vi "Autonomous Independent.vi"   [LabVIEW 2020]
doc: "This VI is called when autonomous begins, and will automatically be terminated when autonomous ends. You can carry out timed or sensor driven robot movement independently without needing to return to the caller."
uses:
  <vilib>/Rock Robotics/WPI/ThirdParty/Phoenix-LabVIEW/Motor Controller/Controls/CTRE_Phoenix_MotorControl_ControlMode.ctl
  <vilib>/Rock Robotics/WPI/Solenoid/WPI_SolenoidValue.ctl
  <vilib>/Rock Robotics/Network Tables/NT Read String.vi
  <vilib>/Rock Robotics/WPI/Utilities/WPI_GetSetVariantRefNum.vi
  <vilib>/Rock Robotics/WPI/RobotDrive/WPI_RobotDriveArcadeDrive_Standard(NoSaturation).vi
  <vilib>/Rock Robotics/WPI/Solenoid/WPI_SolenoidSetEnum.vi
  <vilib>/Rock Robotics/Network Tables/NT Read Number.vi
panel:
  # "Be sure to right-click and choose Data Operations>>Make Current Value default if you want to save the array values with the VI"
types:
  T1 = typedef "WPI_RobotDriveDevRef.ctl" = cluster{"DevStatus":errorcluster, "Motors[]":T2[], "Square Inputs":bool, "Max Output":dbl}
  T2 = typedef "WPI_MotorControlDeviceRef.ctl" = cluster{"DeviceStatus":errorcluster, "Type":T3, "PWM":cluster{"PWM Channel":T4, "DeadBand":T5}, "CAN":cluster{"Device Number":u8, "SetOutput VI Ref":variant, "GetOutput VI Ref":variant, "Enable VI Ref":variant, "Disable VI Ref":variant, "Data":variant}, "Invert":bool, "DIO PWM":cluster{"PWM \"Enable\" Channel":T4, "DIOChannel":T6, "PWM Rate":dbl}}
  T3 = typedef "WPI_MotorControlType.ctl" = enum16{"PWM", "CAN", "DIO PWM"}
  T4 = typedef "FPGA_DIOPWMChannel.ctl" = enum8{"PWM 0", "PWM 1", "PWM 2", "PWM 3", "PWM 4", "PWM 5", "PWM 6", "PWM 7", "PWM 8", "PWM 9", "PWM MXP 0", "PWM MXP 1", "PWM MXP 2", "PWM MXP 3", "PWM MXP 4", "PWM MXP 5", "PWM MXP 6", "PWM MXP 7", "PWM MXP 8", "PWM MXP 9", "Invalid"}
  T5 = typedef "WPI_PWMDeadband.ctl" = cluster{"Name":string, "maxPositivePwm":i32, "minPositivePwm":i32, "centerPwm":i32, "maxNegativePwm":i32, "minNegativePwm":i32, "angularRange":u16}
  T6 = typedef "FPGA_DIOChannel.ctl" = enum8{"DIO 0", "DIO 1", "DIO 2", "DIO 3", "DIO 4", "DIO 5", "DIO 6", "DIO 7", "DIO 8", "DIO 9", "DIO MXP 0", "DIO MXP 1", "DIO MXP 2", "DIO MXP 3", "DIO MXP 4", "DIO MXP 5", "DIO MXP 6", "DIO MXP 7", "DIO MXP 8", "DIO MXP 9", "DIO MXP 10", "DIO MXP 11", "DIO MXP 12", "DIO MXP 13", "DIO MXP 14", "DIO MXP 15", "SPI Port CS1", "SPI Port CS2", "SPI Port CS3", "SPI Port MISO", "SPI Port MOSI", "Invalid"}
  T7 = typedef "WPI_SolenoidDevRef.ctl" = cluster{"DevStatus":errorcluster, "Pneumatics Control Module":u8, "Forward Solenoid Channel":T8, "Reverse Solenoid Channel":T8}
  T8 = typedef "WPI_SolenoidChannel.ctl" = enum8{"Solenoid 0", "Solenoid 1", "Solenoid 2", "Solenoid 3", "Solenoid 4", "Solenoid 5", "Solenoid 6", "Solenoid 7", "Solenoid 8", "Solenoid 9", "Solenoid 10", "Solenoid 11", "Solenoid 12", "Solenoid 13", "Solenoid 14", "Solenoid 15", "Invalid"}
  T9 = typedef "WPI_SolenoidValue.ctl" = enum16{"Off", "On", "Forward", "Reverse"}
  T10 = typedef "CTRE_Phoenix_MotorControl_ControlMode.ctl" = u16
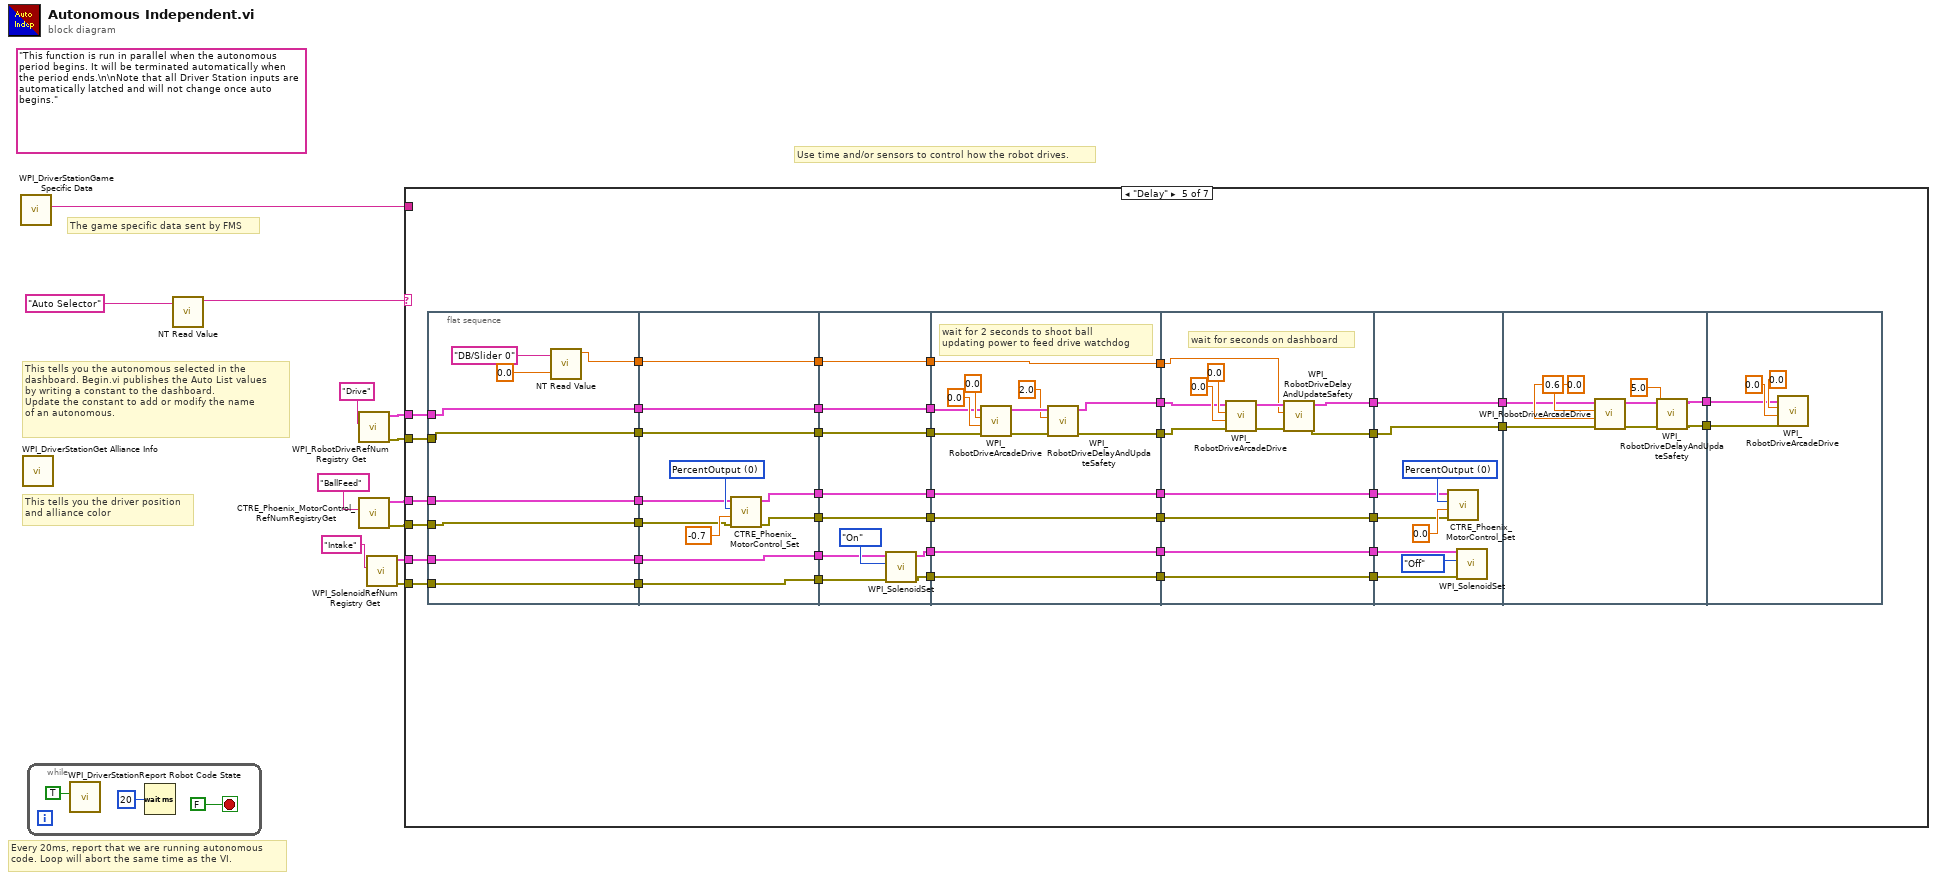
[diagram p0: block diagram]
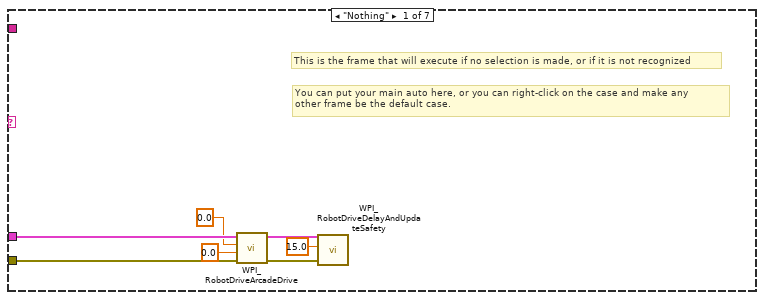
[diagram p2: hidden frame]
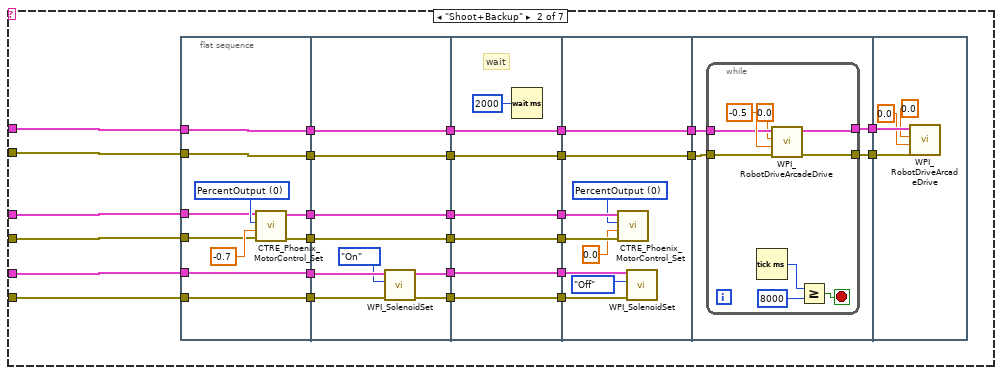
[diagram p3: hidden frame]
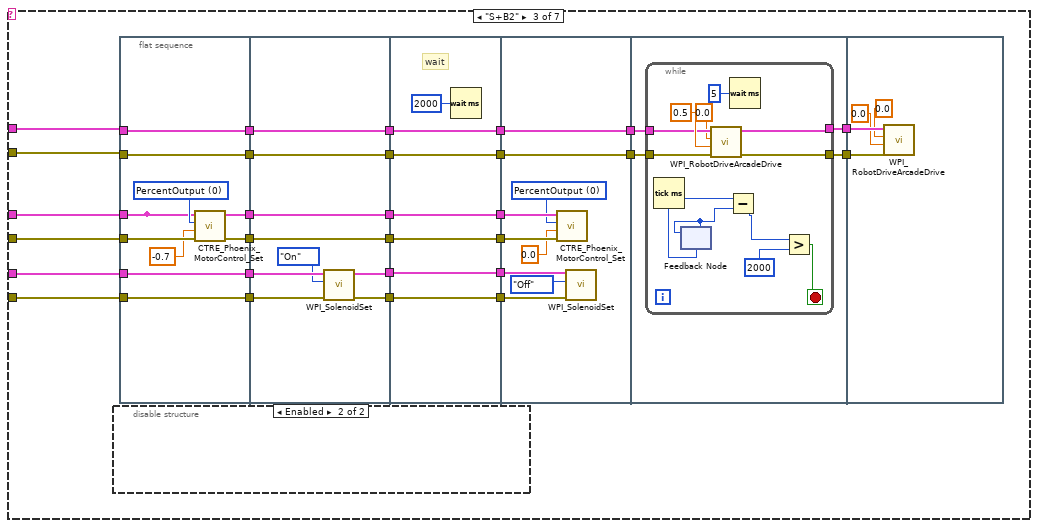
[diagram p4: hidden frame]
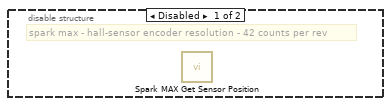
[diagram p5: hidden frame]
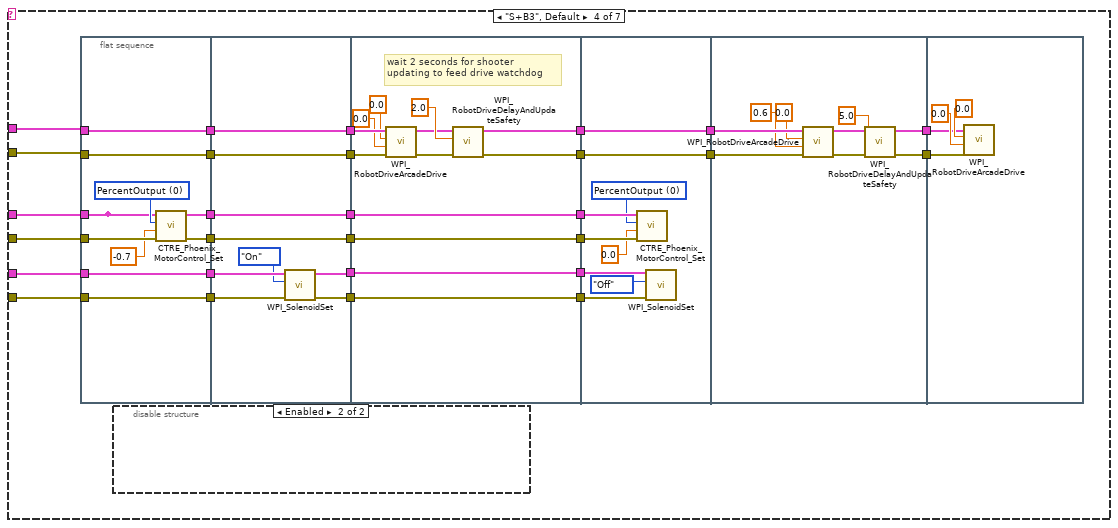
[diagram p6: hidden frame]
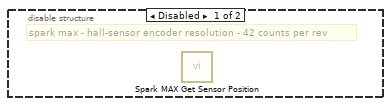
[diagram p7: hidden frame]
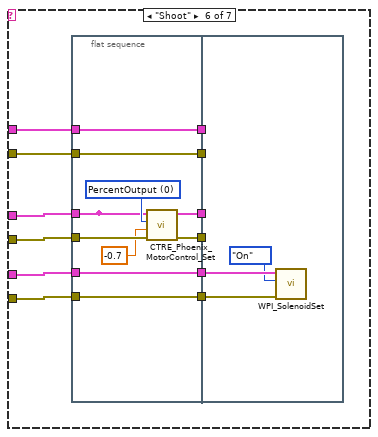
[diagram p8: hidden frame]
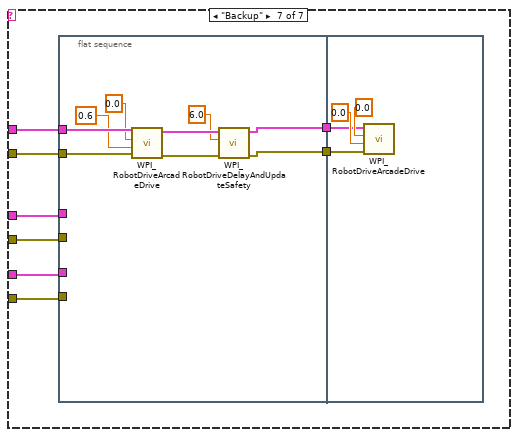
[diagram p9: hidden frame]
diagram:
  (unwired) "This function is run in parallel when the autonomous period begins. It will be terminated automatically when the period ends.\n\nNote that all Driver Station inputs are automatically latched and will not change once auto begins."
  # "The game specific data sent by FMS"
  # "This tells you the autonomous selected in the \ndashboard. Begin.vi publishes the Auto List values\nby writing a constant to the dashboard.\nUpdate the constant to add or modify the name\nof an autonomous."
  # "Every 20ms, report that we are running autonomous\ncode. Loop will abort the same time as the VI."
  # "Use time and/or sensors to control how the robot drives."
  # "This tells you the driver position\nand alliance color"
  n1 = call <vilib>:"WPI_DriverStationGame Specific Data.vi"() -> ("Game Specific Data"=w10:string)  [unwired: 11 in]
  n2 = call <vilib>:"WPI_DriverStationGet Alliance Info.vi"() -> ()  [unwired: 12 out]
  n3 = while {
    stop <- FALSE stop-if-true
    n4 = call <vilib>:"WPI_DriverStationReport Robot Code State.vi"("Autonomous"=TRUE) -> ()  [unwired: 10 in, 1 out]
    n5 = Wait (ms)(milliseconds to wait=u32 20) -> ()  [unwired: 1 out]
  }
  n6 = call-poly <vilib>:"NT Read Value.vi"("Name"="Auto Selector") -> ("String"=w11:string)  [unwired: 9 in, 1 out]
  n7 = call <vilib>:"WPI_RobotDriveRefNum Registry Get.vi"("refnum name"="Drive") -> ("error out"=w8:errorcluster, "RobotDriveDevRef"=w7:T1)  [unwired: 9 in]
  n8 = call <vilib>:"CTRE_Phoenix_MotorControl_RefNumRegistryGet.vi"("refnum name"="BallFeed") -> ("error out"=w2:errorcluster, "PhoenixMotorControlDevRef"=w1:T2)  [unwired: 9 in]
  n9 = call <vilib>:"WPI_SolenoidRefNum Registry Get.vi"("refnum name"="Intake") -> ("error out"=w4:errorcluster, "SolenoidDevRef"=w3:T7)  [unwired: 9 in]
  n10 = case shown="\"Delay\"" w11 {
    tunnel: w10 -> [_ _ _ _ _ _ _]
    tunnel: w8 -> [w21 w36 w107 w192 w294 w395 w422]
    tunnel: w7 -> [w22 w31 w108 w193 w301 w396 w423]
    tunnel: w4 -> [_ w26 w103 w188 w303 w391 w418]
    tunnel: w3 -> [_ w25 w104 w189 w306 w392 w419]
    tunnel: w2 -> [_ w24 w105 w190 w309 w393 w420]
    tunnel: w1 -> [_ w23 w106 w191 w310 w394 w421]
    frame "Nothing" {
      # "You can put your main auto here, or you can right-click on the case and make any\nother frame be the default case."
      # "This is the frame that will execute if no selection is made, or if it is not recognized"
      n11 = call-poly <vilib>:"WPI_RobotDriveArcadeDrive.vi"("error in (no error)"=w21, "Y axis value"=0.0, "X axis value"=0.0, "RobotDriveDevRef"=w22) -> ("error out"=w19:errorcluster, "RobotDriveDevRef"=w20:T1)  [unwired: 5 in, 1 out]
      n12 = call <vilib>:"WPI_RobotDriveDelayAndUpdateSafety.vi"("error in (no error)"=w19, "Delay (s)"=15.0, "RobotDriveDevRef"=w20) -> ()  [unwired: 7 in, 2 out]
    }
    frame "Shoot+Backup" {
      n13 = flat-sequence {
        tunnel: [w53] -> w50
        tunnel: [w54] -> w49
        tunnel: [w58] -> w46
        tunnel: [w57] -> w39
        tunnel: w36 -> [w56]
        tunnel: [w56] -> w35
        tunnel: w31 -> [w55]
        tunnel: [w55] -> w30
        tunnel: w26 -> [w54]
        tunnel: w25 -> [w53]
        tunnel: w24 -> [w52]
        tunnel: w23 -> [w51]
        tunnel: w50 -> [w69]
        tunnel: w49 -> [w68]
        tunnel: [w66] -> w47
        tunnel: w46 -> [w66]
        tunnel: [w65] -> w44
        tunnel: [w64] -> w42
        tunnel: [w63] -> w40
        tunnel: w39 -> [w63]
        tunnel: w35 -> [w62]
        tunnel: [w62] -> w34
        tunnel: w30 -> [w61]
        tunnel: [w61] -> w27
        tunnel: [w75] -> w48
        tunnel: w47 -> [w75]
        tunnel: [w74] -> w45
        tunnel: w44 -> [w74]
        tunnel: [w73] -> w43
        tunnel: w42 -> [w73]
        tunnel: [w72] -> w41
        tunnel: w40 -> [w72]
        tunnel: w34 -> [w71]
        tunnel: [w71] -> w32
        tunnel: [w70] -> w28
        tunnel: w27 -> [w70]
        tunnel: w48 -> [w85]
        tunnel: w45 -> [w83]
        tunnel: w43 -> [w84]
        tunnel: w41 -> [w82]
        tunnel: [w78] -> w33
        tunnel: w32 -> [w78]
        tunnel: [w77] -> w29
        tunnel: w28 -> [w77]
        tunnel: [w89] -> w38
        tunnel: [w88] -> w37
        tunnel: w33 -> [w87]
        tunnel: w29 -> [w86]
        tunnel: w38 -> [w102]
        tunnel: w37 -> [w101]
        frame #0 {
          w60 = T10 0 items=["PercentOutput"=0, "Position"=1, "Velocity"=2, "Current"=3, "Follower"=5, "MotionProfile"=6, "MotionMagic"=7, "MotionProfileArc"=10, "Disabled"=15] ("Control Mode")
          n14 = call <vilib>:"CTRE_Phoenix_MotorControl_Set.vi"("error in (no error)"=w52, "Output"=-0.7, "Control Mode"=w60, "PhoenixMotorControlDevRef"=w51) -> ("error out"=w57:errorcluster, "PhoenixMotorControlDevRef"=w58:T2)  [unwired: 6 in]
        }
        frame #1 {
          n15 = call-poly <vilib>:"WPI_SolenoidSet.vi"("error in (no error)"=w68, "Value"=WPI_SolenoidValue."On", "SolenoidDevRef"=w69) -> ("error out"=w64:errorcluster, "SolenoidDevRef"=w65:T7)  [unwired: 7 in]
        }
        frame #2 {
          # "wait"
          n16 = Wait (ms)(milliseconds to wait=u32 2000) -> ()  [unwired: 1 out]
        }
        frame #3 {
          w81 = T10 0 items=["PercentOutput"=0, "Position"=1, "Velocity"=2, "Current"=3, "Follower"=5, "MotionProfile"=6, "MotionMagic"=7, "MotionProfileArc"=10, "Disabled"=15] ("Control Mode")
          n17 = call <vilib>:"CTRE_Phoenix_MotorControl_Set.vi"("error in (no error)"=w82, "Output"=0.0, "Control Mode"=w81, "PhoenixMotorControlDevRef"=w85) -> ()  [unwired: 6 in, 2 out]
          n18 = call-poly <vilib>:"WPI_SolenoidSet.vi"("error in (no error)"=w84, "Value"=WPI_SolenoidValue."Off", "SolenoidDevRef"=w83) -> ()  [unwired: 7 in, 2 out]
        }
        frame #4 {
          n19 = while {
            tunnel: w86 -> [w94]
            tunnel: w87 -> [w93]
            tunnel: [w91] -> w89
            tunnel: [w90] -> w88
            stop <- w98 stop-if-true
            n20 = Tick Count (ms)() -> (millisecond timer value=w97:u32)
            n21 = call-poly <vilib>:"WPI_RobotDriveArcadeDrive.vi"("error in (no error)"=w93, "Y axis value"=-0.5, "X axis value"=0.0, "RobotDriveDevRef"=w94) -> ("error out"=w90:errorcluster, "RobotDriveDevRef"=w91:T1)  [unwired: 5 in, 1 out]
            n22 = Greater Or Equal?(x=w97, y=u32 8000) -> (x >= y?=w98:bool)
          }
        }
        frame #5 {
          n23 = call-poly <vilib>:"WPI_RobotDriveArcadeDrive.vi"("error in (no error)"=w101, "Y axis value"=0.0, "X axis value"=0.0, "RobotDriveDevRef"=w102) -> ()  [unwired: 5 in, 3 out]
        }
      }
    }
    frame "S+B2" {
      n24 = disable-structure shown="Enabled" {
        frame Disabled {
          # "spark max - hall-sensor encoder resolution - 42 counts per rev"
          n25 = call <vilib>:"Spark MAX Get Sensor Position.vi"() -> ()  [unwired: 8 in, 4 out]
        }
        frame Enabled {
        }
      }
      n26 = flat-sequence {
        tunnel: [w131] -> _
        tunnel: w105 -> [w140]
        tunnel: [w137] -> w130
        tunnel: w104 -> [w137]
        tunnel: [w136] -> w129
        tunnel: w103 -> [w136]
        tunnel: [w135] -> w128
        tunnel: [w134] -> w127
        tunnel: [w133] -> w126
        tunnel: w108 -> [w133]
        tunnel: [w132] -> w125
        tunnel: w107 -> [w132]
        tunnel: w106 -> [w131]
        tunnel: w130 -> [w149]
        tunnel: w129 -> [w148]
        tunnel: [w146] -> w124
        tunnel: w128 -> [w146]
        tunnel: [w145] -> w123
        tunnel: [w144] -> w122
        tunnel: [w143] -> w121
        tunnel: w127 -> [w143]
        tunnel: w126 -> [w142]
        tunnel: [w142] -> w120
        tunnel: w125 -> [w141]
        tunnel: [w141] -> w119
        tunnel: [w155] -> w118
        tunnel: w124 -> [w155]
        tunnel: [w154] -> w117
        tunnel: w123 -> [w154]
        tunnel: [w153] -> w116
        tunnel: w122 -> [w153]
        tunnel: [w152] -> w115
        tunnel: w121 -> [w152]
        tunnel: [w151] -> w114
        tunnel: w120 -> [w151]
        tunnel: [w150] -> w113
        tunnel: w119 -> [w150]
        tunnel: w118 -> [w165]
        tunnel: w117 -> [w163]
        tunnel: w116 -> [w164]
        tunnel: w115 -> [w162]
        tunnel: [w158] -> w112
        tunnel: w114 -> [w158]
        tunnel: w113 -> [w157]
        tunnel: [w157] -> w111
        tunnel: w112 -> [w169]
        tunnel: w111 -> [w168]
        tunnel: [w167] -> w110
        tunnel: [w166] -> w109
        tunnel: w110 -> [w185]
        tunnel: w109 -> [w184]
        frame #0 {
          w139 = T10 0 items=["PercentOutput"=0, "Position"=1, "Velocity"=2, "Current"=3, "Follower"=5, "MotionProfile"=6, "MotionMagic"=7, "MotionProfileArc"=10, "Disabled"=15] ("Control Mode")
          n27 = call <vilib>:"CTRE_Phoenix_MotorControl_Set.vi"("error in (no error)"=w140, "Output"=-0.7, "Control Mode"=w139, "PhoenixMotorControlDevRef"=w131) -> ("error out"=w134:errorcluster, "PhoenixMotorControlDevRef"=w135:T2)  [unwired: 6 in]
        }
        frame #1 {
          n28 = call-poly <vilib>:"WPI_SolenoidSet.vi"("error in (no error)"=w148, "Value"=WPI_SolenoidValue."On", "SolenoidDevRef"=w149) -> ("error out"=w144:errorcluster, "SolenoidDevRef"=w145:T7)  [unwired: 7 in]
        }
        frame #2 {
          # "wait"
          n29 = Wait (ms)(milliseconds to wait=u32 2000) -> ()  [unwired: 1 out]
        }
        frame #3 {
          w161 = T10 0 items=["PercentOutput"=0, "Position"=1, "Velocity"=2, "Current"=3, "Follower"=5, "MotionProfile"=6, "MotionMagic"=7, "MotionProfileArc"=10, "Disabled"=15] ("Control Mode")
          n30 = call <vilib>:"CTRE_Phoenix_MotorControl_Set.vi"("error in (no error)"=w162, "Output"=0.0, "Control Mode"=w161, "PhoenixMotorControlDevRef"=w165) -> ()  [unwired: 6 in, 2 out]
          n31 = call-poly <vilib>:"WPI_SolenoidSet.vi"("error in (no error)"=w164, "Value"=WPI_SolenoidValue."Off", "SolenoidDevRef"=w163) -> ()  [unwired: 7 in, 2 out]
        }
        frame #4 {
          n32 = while {
            tunnel: w169 -> [w180]
            tunnel: w168 -> [w179]
            tunnel: [w177] -> w167
            tunnel: [w176] -> w166
            stop <- w171 stop-if-true
            n33 = Tick Count (ms)() -> (millisecond timer value=w174:u32)
            n34 = feedback #1(w174) -> (w175:u32)
            n35 = feedback-in #1(w175) -> ()
            n36 = call-poly <vilib>:"WPI_RobotDriveArcadeDrive.vi"("error in (no error)"=w179, "Y axis value"=0.5, "X axis value"=0.0, "RobotDriveDevRef"=w180) -> ("error out"=w176:errorcluster, "RobotDriveDevRef"=w177:T1)  [unwired: 5 in, 1 out]
            n37 = Subtract(x=w174, y=w175) -> (x-y=w172:u32)
            n38 = Wait (ms)(milliseconds to wait=u32 5) -> ()  [unwired: 1 out]
            n39 = Greater?(x=w172, y=u32 2000) -> (0:w171:bool)
          }
        }
        frame #5 {
          n40 = call-poly <vilib>:"WPI_RobotDriveArcadeDrive.vi"("error in (no error)"=w184, "Y axis value"=0.0, "X axis value"=0.0, "RobotDriveDevRef"=w185) -> ()  [unwired: 5 in, 3 out]
        }
      }
    }
    frame "S+B3", Default {
      n41 = flat-sequence {
        tunnel: [w214] -> _
        tunnel: w190 -> [w223]
        tunnel: [w220] -> w213
        tunnel: w189 -> [w220]
        tunnel: [w219] -> w212
        tunnel: w188 -> [w219]
        tunnel: [w218] -> w211
        tunnel: [w217] -> w210
        tunnel: [w216] -> w209
        tunnel: w193 -> [w216]
        tunnel: [w215] -> w208
        tunnel: w192 -> [w215]
        tunnel: w191 -> [w214]
        tunnel: w213 -> [w232]
        tunnel: w212 -> [w231]
        tunnel: [w229] -> w207
        tunnel: w211 -> [w229]
        tunnel: [w228] -> w206
        tunnel: [w227] -> w205
        tunnel: [w226] -> w204
        tunnel: w210 -> [w226]
        tunnel: w209 -> [w225]
        tunnel: [w225] -> w203
        tunnel: w208 -> [w224]
        tunnel: [w224] -> w202
        tunnel: [w245] -> w201
        tunnel: w207 -> [w245]
        tunnel: [w244] -> w200
        tunnel: w206 -> [w244]
        tunnel: [w243] -> w199
        tunnel: w205 -> [w243]
        tunnel: [w242] -> w198
        tunnel: w204 -> [w242]
        tunnel: [w236] -> w197
        tunnel: w203 -> [w238]
        tunnel: [w235] -> w196
        tunnel: w202 -> [w237]
        tunnel: w201 -> [w254]
        tunnel: w200 -> [w252]
        tunnel: w199 -> [w253]
        tunnel: w198 -> [w251]
        tunnel: [w247] -> w195
        tunnel: w197 -> [w247]
        tunnel: w196 -> [w246]
        tunnel: [w246] -> w194
        tunnel: w195 -> [w263]
        tunnel: w194 -> [w262]
        tunnel: [w257] -> w187
        tunnel: [w256] -> w186
        tunnel: w187 -> [w265]
        tunnel: w186 -> [w264]
        frame #0 {
          w222 = T10 0 items=["PercentOutput"=0, "Position"=1, "Velocity"=2, "Current"=3, "Follower"=5, "MotionProfile"=6, "MotionMagic"=7, "MotionProfileArc"=10, "Disabled"=15] ("Control Mode")
          n42 = call <vilib>:"CTRE_Phoenix_MotorControl_Set.vi"("error in (no error)"=w223, "Output"=-0.7, "Control Mode"=w222, "PhoenixMotorControlDevRef"=w214) -> ("error out"=w217:errorcluster, "PhoenixMotorControlDevRef"=w218:T2)  [unwired: 6 in]
        }
        frame #1 {
          n43 = call-poly <vilib>:"WPI_SolenoidSet.vi"("error in (no error)"=w231, "Value"=WPI_SolenoidValue."On", "SolenoidDevRef"=w232) -> ("error out"=w227:errorcluster, "SolenoidDevRef"=w228:T7)  [unwired: 7 in]
        }
        frame #2 {
          # "wait 2 seconds for shooter\nupdating to feed drive watchdog"
          n44 = call-poly <vilib>:"WPI_RobotDriveArcadeDrive.vi"("error in (no error)"=w237, "Y axis value"=0.0, "X axis value"=0.0, "RobotDriveDevRef"=w238) -> ("error out"=w240:errorcluster, "RobotDriveDevRef"=w239:T1)  [unwired: 5 in, 1 out]
          n45 = call <vilib>:"WPI_RobotDriveDelayAndUpdateSafety.vi"("error in (no error)"=w240, "Delay (s)"=2.0, "RobotDriveDevRef"=w239) -> ("error out"=w235:errorcluster, "RobotDriveDevRef 2"=w236:T1)  [unwired: 7 in]
        }
        frame #3 {
          w250 = T10 0 items=["PercentOutput"=0, "Position"=1, "Velocity"=2, "Current"=3, "Follower"=5, "MotionProfile"=6, "MotionMagic"=7, "MotionProfileArc"=10, "Disabled"=15] ("Control Mode")
          n46 = call <vilib>:"CTRE_Phoenix_MotorControl_Set.vi"("error in (no error)"=w251, "Output"=0.0, "Control Mode"=w250, "PhoenixMotorControlDevRef"=w254) -> ()  [unwired: 6 in, 2 out]
          n47 = call-poly <vilib>:"WPI_SolenoidSet.vi"("error in (no error)"=w253, "Value"=WPI_SolenoidValue."Off", "SolenoidDevRef"=w252) -> ()  [unwired: 7 in, 2 out]
        }
        frame #4 {
          n48 = call-poly <vilib>:"WPI_RobotDriveArcadeDrive.vi"("error in (no error)"=w262, "Y axis value"=0.6, "X axis value"=0.0, "RobotDriveDevRef"=w263) -> ("error out"=w258:errorcluster, "RobotDriveDevRef"=w259:T1)  [unwired: 5 in, 1 out]
          n49 = call <vilib>:"WPI_RobotDriveDelayAndUpdateSafety.vi"("error in (no error)"=w258, "Delay (s)"=5.0, "RobotDriveDevRef"=w259) -> ("error out"=w256:errorcluster, "RobotDriveDevRef 2"=w257:T1)  [unwired: 7 in]
        }
        frame #5 {
          n50 = call-poly <vilib>:"WPI_RobotDriveArcadeDrive.vi"("error in (no error)"=w264, "Y axis value"=0.0, "X axis value"=0.0, "RobotDriveDevRef"=w265) -> ()  [unwired: 5 in, 3 out]
        }
      }
      n51 = disable-structure shown="Enabled" {
        frame Disabled {
          # "spark max - hall-sensor encoder resolution - 42 counts per rev"
          n52 = call <vilib>:"Spark MAX Get Sensor Position.vi"() -> ()  [unwired: 8 in, 4 out]
        }
        frame Enabled {
        }
      }
    }
    frame "Delay" {
      n53 = flat-sequence {
        tunnel: [w320] -> w311
        tunnel: w310 -> [w320]
        tunnel: w309 -> [w319]
        tunnel: [w319] -> w308
        tunnel: [w318] -> w307
        tunnel: w306 -> [w318]
        tunnel: [w317] -> w304
        tunnel: w303 -> [w317]
        tunnel: w301 -> [w314]
        tunnel: [w314] -> w298
        tunnel: [w313] -> w295
        tunnel: w294 -> [w313]
        tunnel: [w312] -> w283
        tunnel: w311 -> [w329]
        tunnel: w308 -> [w328]
        tunnel: w307 -> [w327]
        tunnel: [w327] -> w305
        tunnel: w304 -> [w326]
        tunnel: [w326] -> w302
        tunnel: [w325] -> w299
        tunnel: w298 -> [w325]
        tunnel: [w324] -> w296
        tunnel: w295 -> [w324]
        tunnel: [w323] -> w292
        tunnel: [w322] -> w290
        tunnel: [w321] -> w284
        tunnel: w283 -> [w321]
        tunnel: w305 -> [w340]
        tunnel: w302 -> [w339]
        tunnel: [w338] -> w300
        tunnel: w299 -> [w338]
        tunnel: [w337] -> w297
        tunnel: w296 -> [w337]
        tunnel: [w336] -> w293
        tunnel: w292 -> [w336]
        tunnel: [w335] -> w291
        tunnel: w290 -> [w335]
        tunnel: [w334] -> w289
        tunnel: [w333] -> w288
        tunnel: [w332] -> w285
        tunnel: w284 -> [w332]
        tunnel: w300 -> [w351]
        tunnel: w297 -> [w350]
        tunnel: [w349] -> w282
        tunnel: w293 -> [w349]
        tunnel: [w348] -> w280
        tunnel: w291 -> [w348]
        tunnel: [w347] -> w278
        tunnel: w289 -> [w347]
        tunnel: [w346] -> w276
        tunnel: w288 -> [w346]
        tunnel: [w345] -> w274
        tunnel: [w344] -> w272
        tunnel: w285 -> [w342]
        tunnel: [w342] -> w270
        tunnel: w282 -> [w368]
        tunnel: [w368] -> w281
        tunnel: w280 -> [w367]
        tunnel: [w367] -> w279
        tunnel: w278 -> [w366]
        tunnel: [w366] -> w277
        tunnel: w276 -> [w365]
        tunnel: [w365] -> w275
        tunnel: w274 -> [w360]
        tunnel: [w358] -> w273
        tunnel: w272 -> [w359]
        tunnel: [w357] -> w271
        tunnel: w270 -> [w356]
        tunnel: w281 -> [w374]
        tunnel: w279 -> [w373]
        tunnel: w277 -> [w372]
        tunnel: w275 -> [w371]
        tunnel: [w370] -> w287
        tunnel: w273 -> [w370]
        tunnel: w271 -> [w369]
        tunnel: [w369] -> w286
        tunnel: w287 -> [w381]
        tunnel: w286 -> [w380]
        tunnel: [w379] -> w269
        tunnel: [w378] -> w268
        tunnel: w269 -> [w388]
        tunnel: w268 -> [w387]
        frame #0 {
          n54 = call-poly <vilib>:"NT Read Value.vi"("Default Value"=0.0, "Name"="DB/Slider 0") -> ("Numeric"=w312:dbl)  [unwired: 8 in, 1 out]
        }
        frame #1 {
          w331 = T10 0 items=["PercentOutput"=0, "Position"=1, "Velocity"=2, "Current"=3, "Follower"=5, "MotionProfile"=6, "MotionMagic"=7, "MotionProfileArc"=10, "Disabled"=15] ("Control Mode")
          n55 = call <vilib>:"CTRE_Phoenix_MotorControl_Set.vi"("error in (no error)"=w328, "Output"=-0.7, "Control Mode"=w331, "PhoenixMotorControlDevRef"=w329) -> ("error out"=w322:errorcluster, "PhoenixMotorControlDevRef"=w323:T2)  [unwired: 6 in]
        }
        frame #2 {
          n56 = call-poly <vilib>:"WPI_SolenoidSet.vi"("error in (no error)"=w339, "Value"=WPI_SolenoidValue."On", "SolenoidDevRef"=w340) -> ("error out"=w333:errorcluster, "SolenoidDevRef"=w334:T7)  [unwired: 7 in]
        }
        frame #3 {
          # "wait for 2 seconds to shoot ball\nupdating power to feed drive watchdog"
          n57 = call-poly <vilib>:"WPI_RobotDriveArcadeDrive.vi"("error in (no error)"=w350, "Y axis value"=0.0, "X axis value"=0.0, "RobotDriveDevRef"=w351) -> ("error out"=w355:errorcluster, "RobotDriveDevRef"=w354:T1)  [unwired: 5 in, 1 out]
          n58 = call <vilib>:"WPI_RobotDriveDelayAndUpdateSafety.vi"("error in (no error)"=w355, "Delay (s)"=2.0, "RobotDriveDevRef"=w354) -> ("error out"=w344:errorcluster, "RobotDriveDevRef 2"=w345:T1)  [unwired: 7 in]
        }
        frame #4 {
          # "wait for seconds on dashboard"
          n59 = call-poly <vilib>:"WPI_RobotDriveArcadeDrive.vi"("error in (no error)"=w359, "Y axis value"=0.0, "X axis value"=0.0, "RobotDriveDevRef"=w360) -> ("error out"=w364:errorcluster, "RobotDriveDevRef"=w363:T1)  [unwired: 5 in, 1 out]
          n60 = call <vilib>:"WPI_RobotDriveDelayAndUpdateSafety.vi"("error in (no error)"=w364, "Delay (s)"=w356, "RobotDriveDevRef"=w363) -> ("error out"=w357:errorcluster, "RobotDriveDevRef 2"=w358:T1)  [unwired: 7 in]
        }
        frame #5 {
          w377 = T10 0 items=["PercentOutput"=0, "Position"=1, "Velocity"=2, "Current"=3, "Follower"=5, "MotionProfile"=6, "MotionMagic"=7, "MotionProfileArc"=10, "Disabled"=15] ("Control Mode")
          n61 = call <vilib>:"CTRE_Phoenix_MotorControl_Set.vi"("error in (no error)"=w373, "Output"=0.0, "Control Mode"=w377, "PhoenixMotorControlDevRef"=w374) -> ()  [unwired: 6 in, 2 out]
          n62 = call-poly <vilib>:"WPI_SolenoidSet.vi"("error in (no error)"=w371, "Value"=WPI_SolenoidValue."Off", "SolenoidDevRef"=w372) -> ()  [unwired: 7 in, 2 out]
        }
        frame #6 {
          n63 = call-poly <vilib>:"WPI_RobotDriveArcadeDrive.vi"("error in (no error)"=w380, "Y axis value"=0.6, "X axis value"=0.0, "RobotDriveDevRef"=w381) -> ("error out"=w386:errorcluster, "RobotDriveDevRef"=w385:T1)  [unwired: 5 in, 1 out]
          n64 = call <vilib>:"WPI_RobotDriveDelayAndUpdateSafety.vi"("error in (no error)"=w386, "Delay (s)"=5.0, "RobotDriveDevRef"=w385) -> ("error out"=w378:errorcluster, "RobotDriveDevRef 2"=w379:T1)  [unwired: 7 in]
        }
        frame #7 {
          n65 = call-poly <vilib>:"WPI_RobotDriveArcadeDrive.vi"("error in (no error)"=w387, "Y axis value"=0.0, "X axis value"=0.0, "RobotDriveDevRef"=w388) -> ()  [unwired: 5 in, 3 out]
        }
      }
    }
    frame "Shoot" {
      n66 = flat-sequence {
        tunnel: w394 -> [w403]
        tunnel: w393 -> [w412]
        tunnel: [w409] -> w402
        tunnel: w392 -> [w409]
        tunnel: [w408] -> w401
        tunnel: w391 -> [w408]
        tunnel: [w407] -> w400
        tunnel: [w406] -> w399
        tunnel: [w405] -> w398
        tunnel: w396 -> [w405]
        tunnel: [w404] -> w397
        tunnel: w395 -> [w404]
        tunnel: [w403] -> _
        tunnel: w402 -> [w415]
        tunnel: w401 -> [w414]
        tunnel: w400 -> [_]
        tunnel: w399 -> [_]
        tunnel: w398 -> [_]
        tunnel: w397 -> [_]
        frame #0 {
          w411 = T10 0 items=["PercentOutput"=0, "Position"=1, "Velocity"=2, "Current"=3, "Follower"=5, "MotionProfile"=6, "MotionMagic"=7, "MotionProfileArc"=10, "Disabled"=15] ("Control Mode")
          n67 = call <vilib>:"CTRE_Phoenix_MotorControl_Set.vi"("error in (no error)"=w412, "Output"=-0.7, "Control Mode"=w411, "PhoenixMotorControlDevRef"=w403) -> ("error out"=w406:errorcluster, "PhoenixMotorControlDevRef"=w407:T2)  [unwired: 6 in]
        }
        frame #1 {
          n68 = call-poly <vilib>:"WPI_SolenoidSet.vi"("error in (no error)"=w414, "Value"=WPI_SolenoidValue."On", "SolenoidDevRef"=w415) -> ()  [unwired: 7 in, 2 out]
        }
      }
    }
    frame "Backup" {
      n69 = flat-sequence {
        tunnel: w421 -> [_]
        tunnel: w420 -> [_]
        tunnel: w419 -> [_]
        tunnel: w418 -> [_]
        tunnel: w423 -> [w432]
        tunnel: w422 -> [w431]
        tunnel: [w425] -> w417
        tunnel: [w424] -> w416
        tunnel: w417 -> [w434]
        tunnel: w416 -> [w433]
        frame #0 {
          n70 = call-poly <vilib>:"WPI_RobotDriveArcadeDrive.vi"("error in (no error)"=w431, "Y axis value"=0.6, "X axis value"=0.0, "RobotDriveDevRef"=w432) -> ("error out"=w427:errorcluster, "RobotDriveDevRef"=w428:T1)  [unwired: 5 in, 1 out]
          n71 = call <vilib>:"WPI_RobotDriveDelayAndUpdateSafety.vi"("error in (no error)"=w427, "Delay (s)"=6.0, "RobotDriveDevRef"=w428) -> ("error out"=w424:errorcluster, "RobotDriveDevRef 2"=w425:T1)  [unwired: 7 in]
        }
        frame #1 {
          n72 = call-poly <vilib>:"WPI_RobotDriveArcadeDrive.vi"("error in (no error)"=w433, "Y axis value"=0.0, "X axis value"=0.0, "RobotDriveDevRef"=w434) -> ()  [unwired: 5 in, 3 out]
        }
      }
    }
  }
